vi "Q14070Z130主界面.vi"() -> ()   [LabVIEW 2013]
panel:
  out "操作步骤":bool[](array[boolean])
  out "实际涂脂":i32 format="%.0g"
  out "涂脂频率":dbl
  out "涂脂次数":i32
  out "气缸压装":dbl
  out "塞头辅具":dbl
  out "定位辅具":dbl
  out "压装辅具":dbl
  out "拧紧信号":dbl
  out "涂脂启动":dbl
  out "螺栓取料":dbl
  out "弹垫取料":dbl
  out "防尘罩O型圈":dbl
  out "胶塞取料":dbl
  out "J728程序选择":bool
  out "涂脂阀2":bool
  out "涂脂阀1":bool
  out "涂脂按钮2":bool
  out "涂脂按钮1":bool
  out "启动1按钮":bool
  out "启动2按钮":bool
  out "压缸下压时间":dbl
  out "扫描条码完成":bool
  out "扫描条码触发":bool
  out "开始时间":string
  in  "结束时间":string
  in  "返工次数":i32
  out "J706程序选择":bool
  out "J709程序选择":bool
  in  "产品ID":string
  out "员工ID":string
  out "员工姓名":string
  out "参数保存错误":errorcluster
  in  "报警清除":bool
  in  "参数加载":bool
  in  "型号选择":u32(ring) items=["J706", "J709", "J728", "J728A", "J728B", "J506X"]
  out "参数加载错误":errorcluster
  in  "停止":bool
  out "ADODB._Connection Out":refnum<k7>
  out "参数查询错误":errorcluster
  in  "联线按钮":bool
  out "通讯状态":bool
  in  "选项卡控件":enum32{"自动界面", "物料批次号输入", "参数查询"}(tab)
  out "涂脂报警工步号":u32 caption="工步号1"
  out "自动工步提示 3":string
  out "J728工布号提示":string
  in  "J728工步号提示":i32
  in  "产品ID字符位数":dbl
  in  "批次号工步号":u32=5 caption="工步号1"
  out "压装辅具在位":bool
  out "定位辅具在位":bool
  out "塞头辅具在位":bool
  out "记号笔在位":bool
  out "取压装辅具指示灯":bool
  out "取定位辅具指示灯":bool
  out "取塞头辅具指示灯":bool
  out "取记号笔指示灯":bool
  out "涂脂阀3":bool
  out "绿灯":bool
  out "黄灯":bool
  out "红灯":bool
  out "涂脂按钮3":bool
  in  "J709工步号提示":u32 caption="工步号1"
  out "自动工步提示 2":string
  out "自动工步号":u32 caption="工步号1"
  in  "报警工步号":u32 caption="工步号1"
  out "自动工步提示":string
  out "报警提示":string
  out "安全光幕":bool
  out "急停按钮":bool
  out "复位按钮":bool
  out "手动/自动":bool
  in  "压装气缸下降":bool
  in  "压装气缸上升":bool
  out "压装气缸上位检测":bool
  out "压装气缸下位检测":bool
  out "压装气缸下压阀":bool
  out "上序合格":bool
  out "上序完成":bool
  out "本序完成":bool
  out "本序合格":bool
  in  "装防尘罩循环启动":bool
  out "批次号提示":string
  in  "弹垫批次号位数":dbl
  in  "花键套批次号位数":dbl
  in  "胶塞批次号位数":dbl
  in  "螺栓批次号位数":dbl
  in  "防尘罩批次号位数":dbl
  out "弹垫批次号输入成功":bool
  out "花键套批次号输入成功":bool
  out "胶塞批次号输入成功":bool
  out "螺栓批次号输入成功":bool
  out "防尘罩批次号输入成功":bool
  in  "弹垫批次号":string
  in  "花键套批次号":string
  in  "胶塞批次号":string
  in  "螺栓批次号":string
  in  "防尘罩批次号":string
  in  "参数保存":bool
  in  "参数查询":bool
  in  "参数列表":string[][](table)
  # "装防尘罩"
  # "Copying (C) 2015 湖北唯思凌科装备制造有限公司 版权所有"
  # "输入成功"
  # "批次号位数"
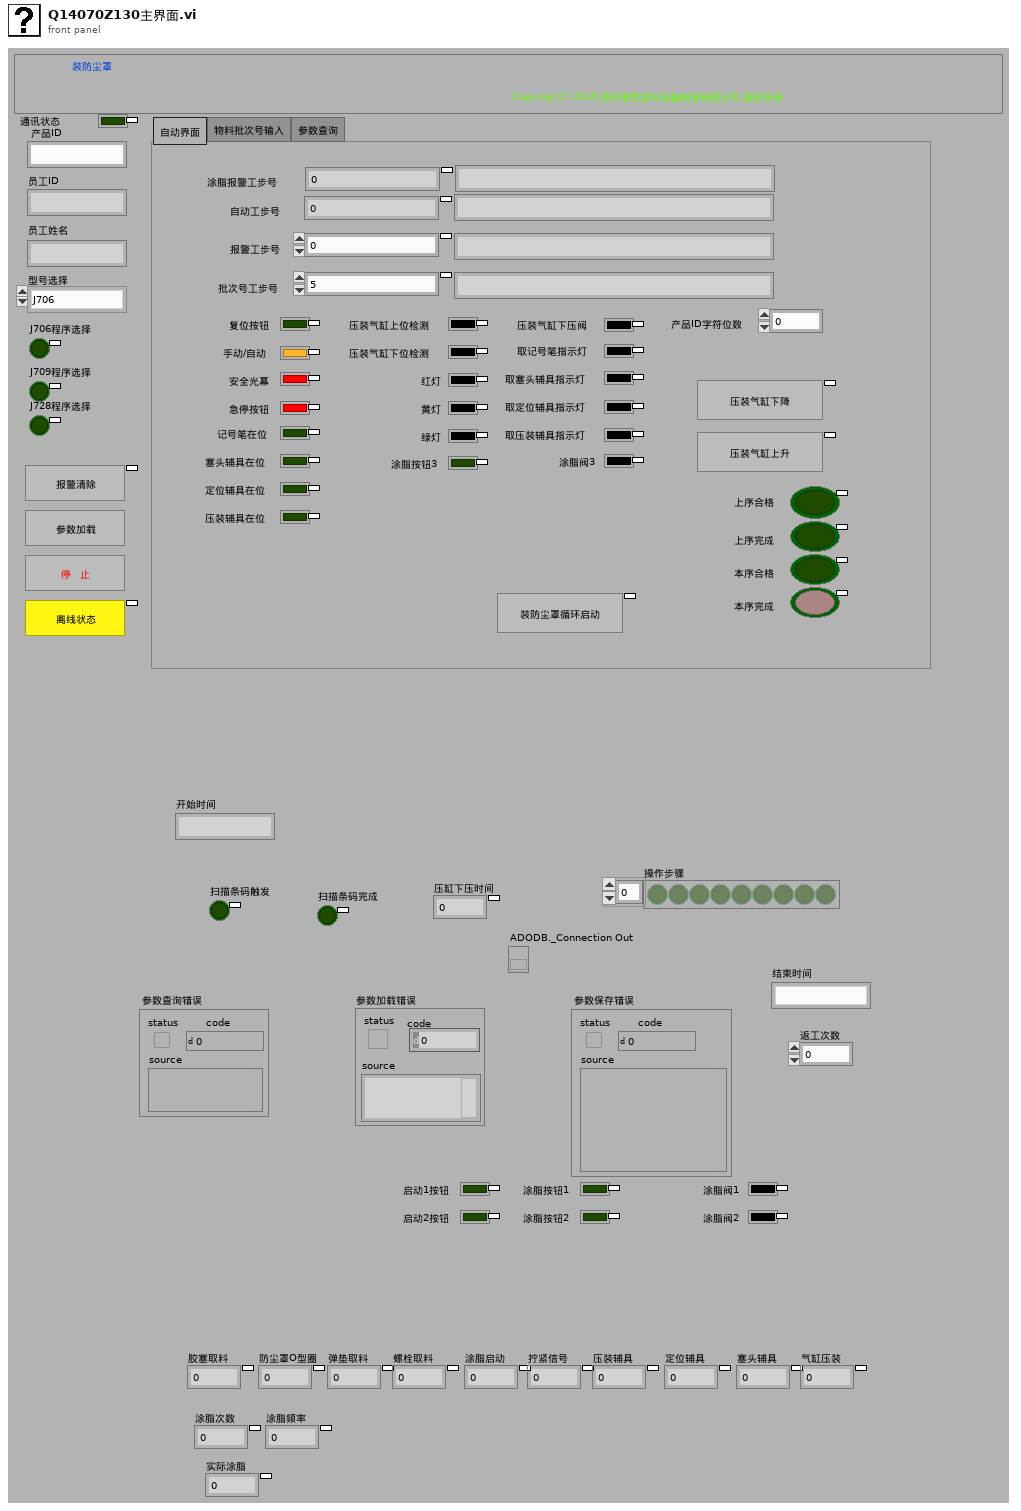
[diagram p1: front panel]
types:
  T1 = enum32{"invalid app kind", "Development System", "Run Time System", "Student Edition", "Embedded LabVIEW", "Evaluation", "Custom"}
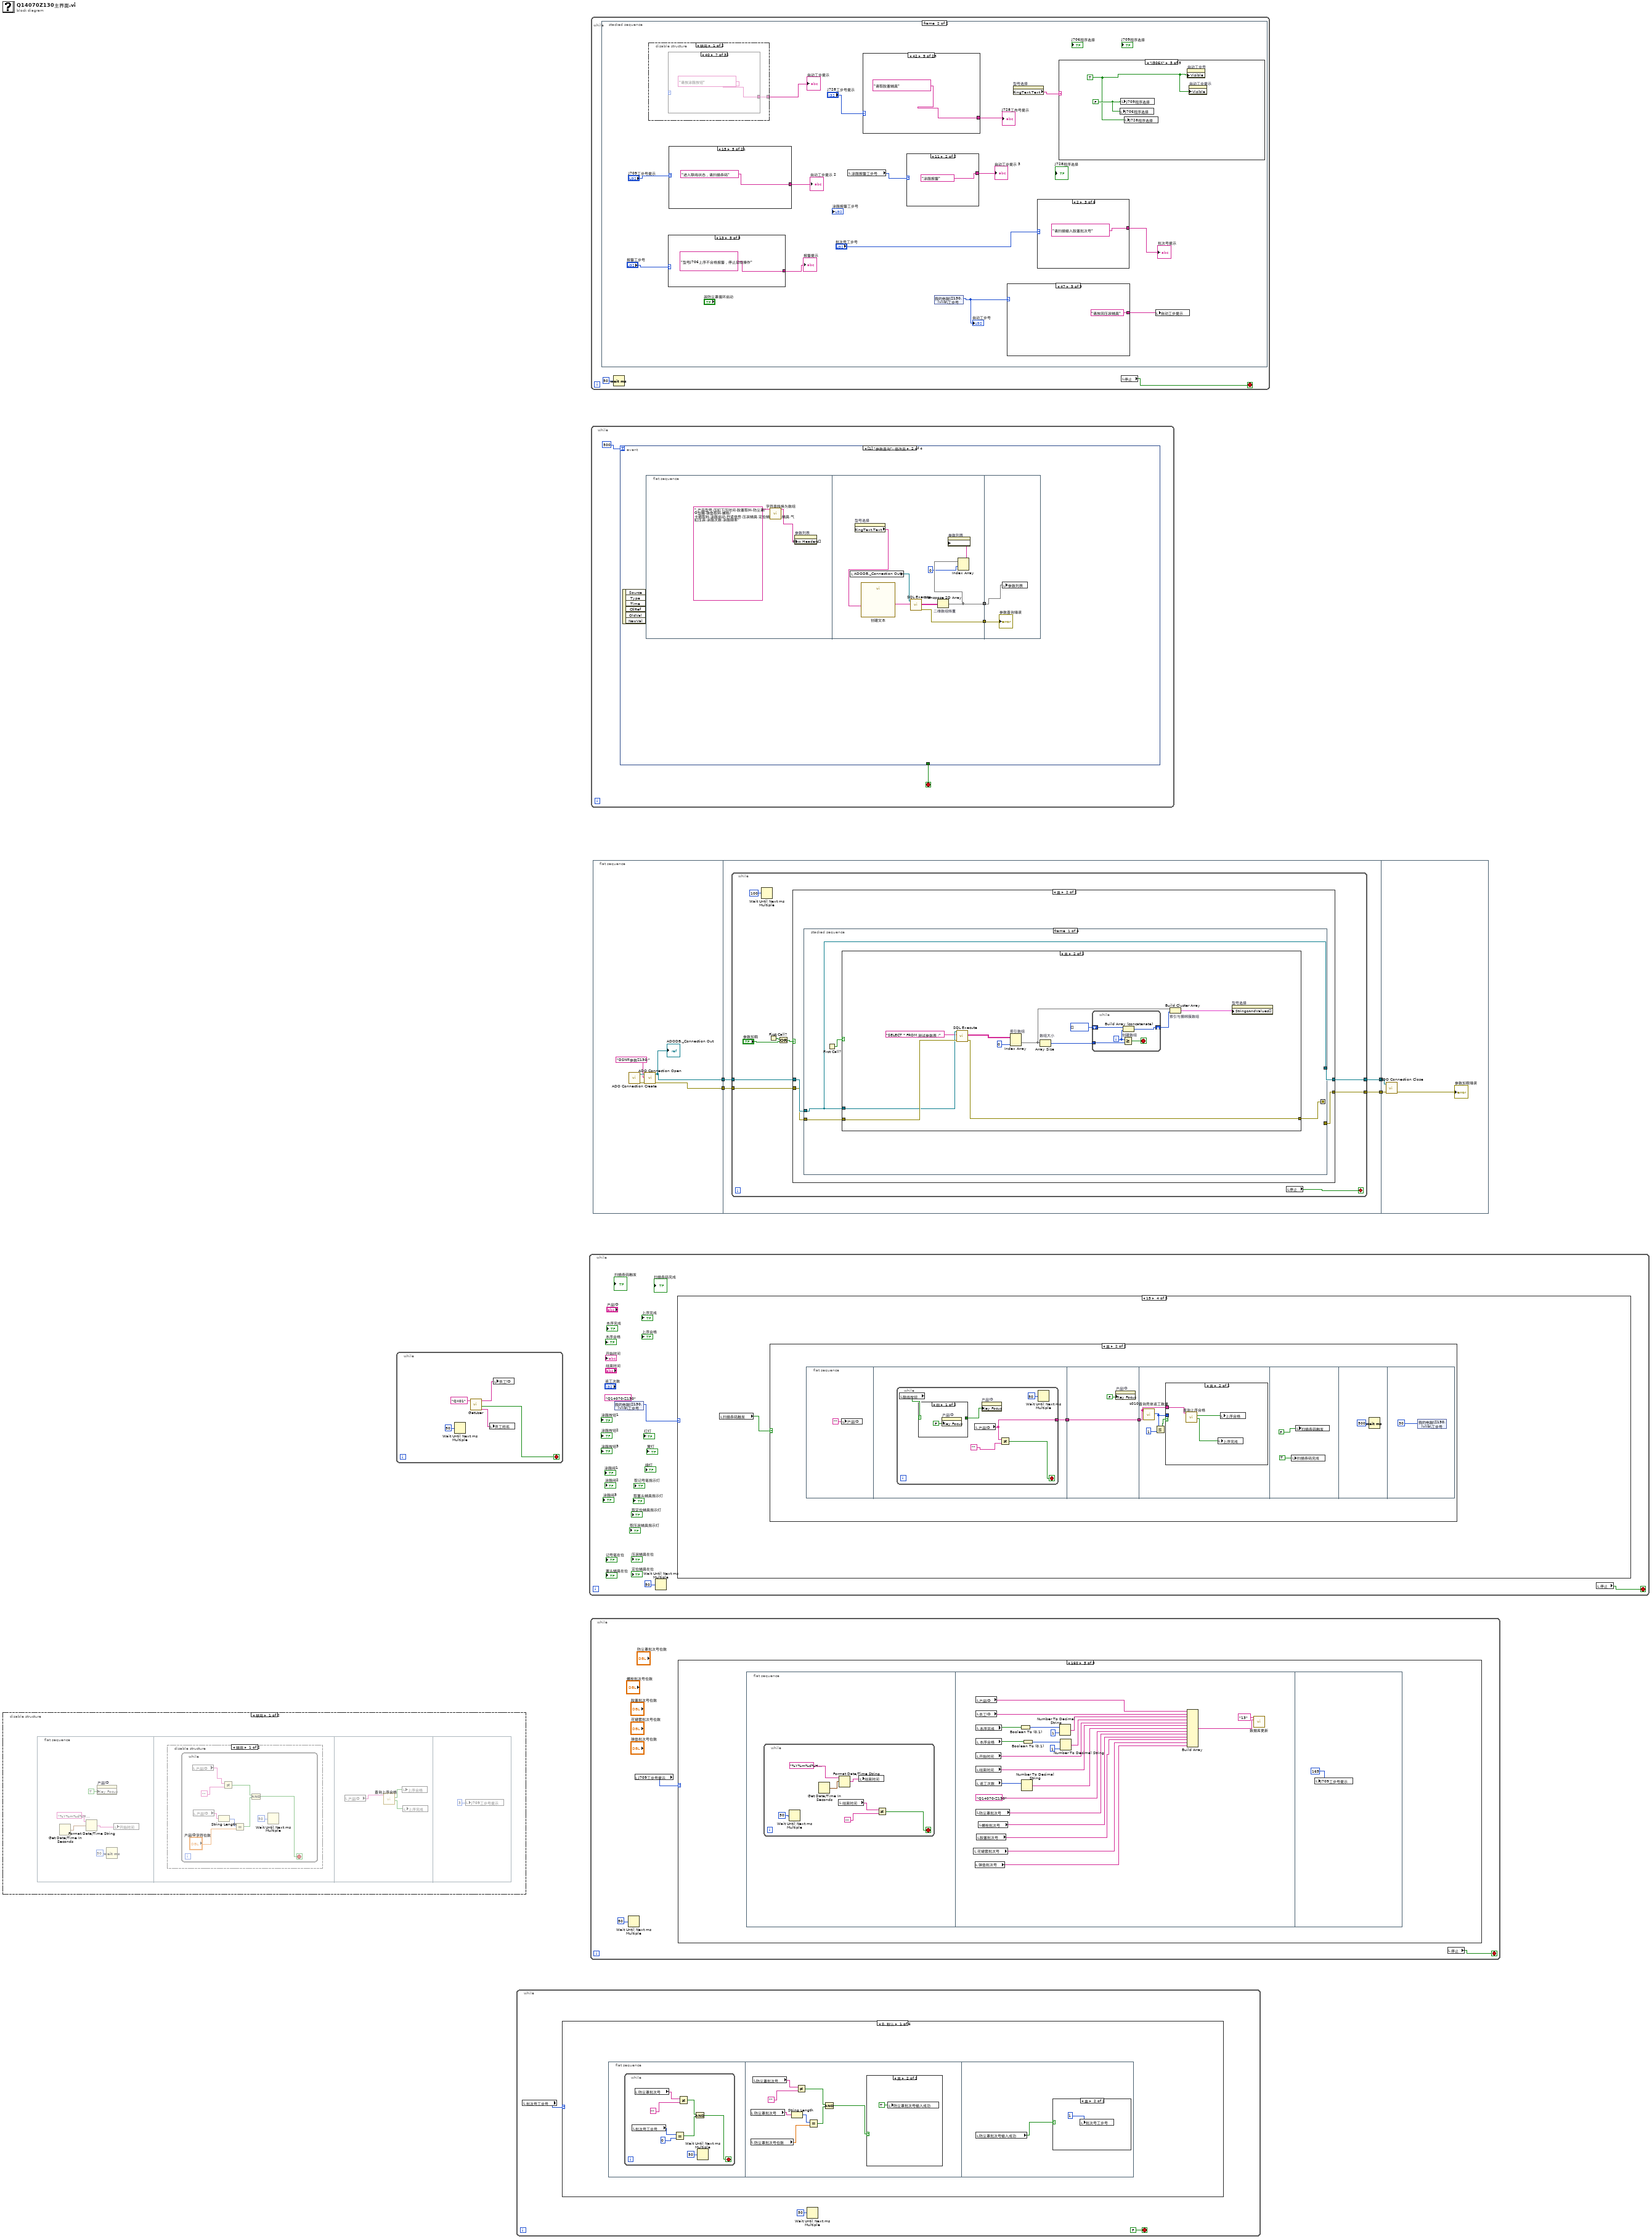
[diagram p0: block diagram]
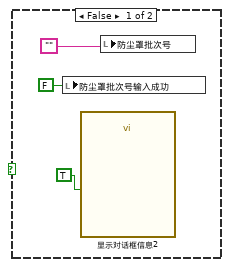
[diagram p4: hidden frame]
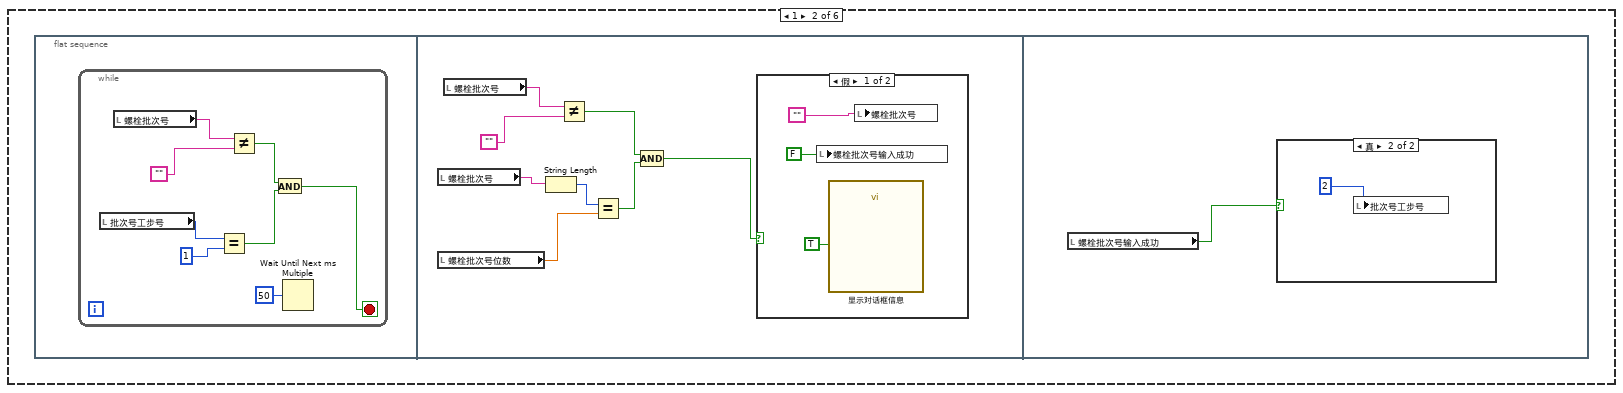
[diagram p6: hidden frame]
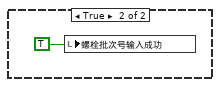
[diagram p7: hidden frame]
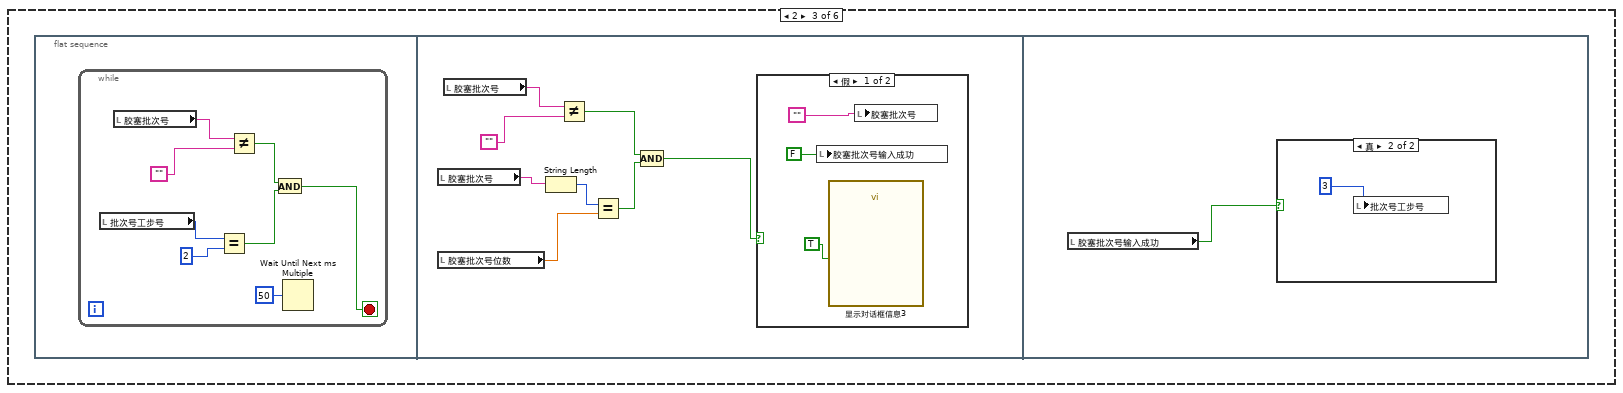
[diagram p9: hidden frame]
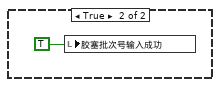
[diagram p10: hidden frame]
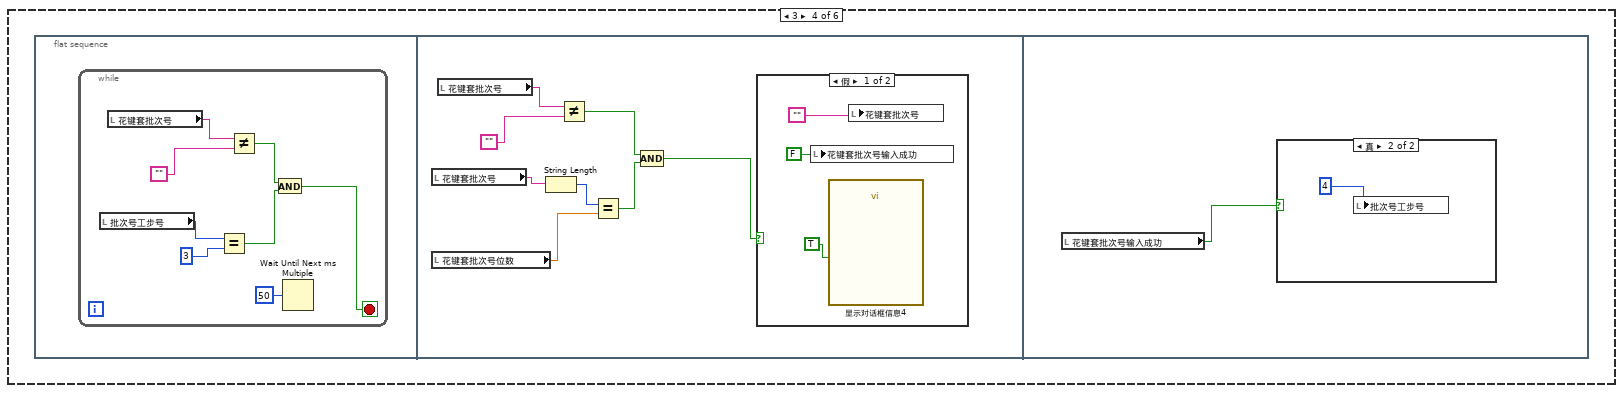
[diagram p12: hidden frame]
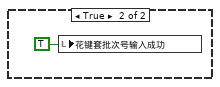
[diagram p13: hidden frame]
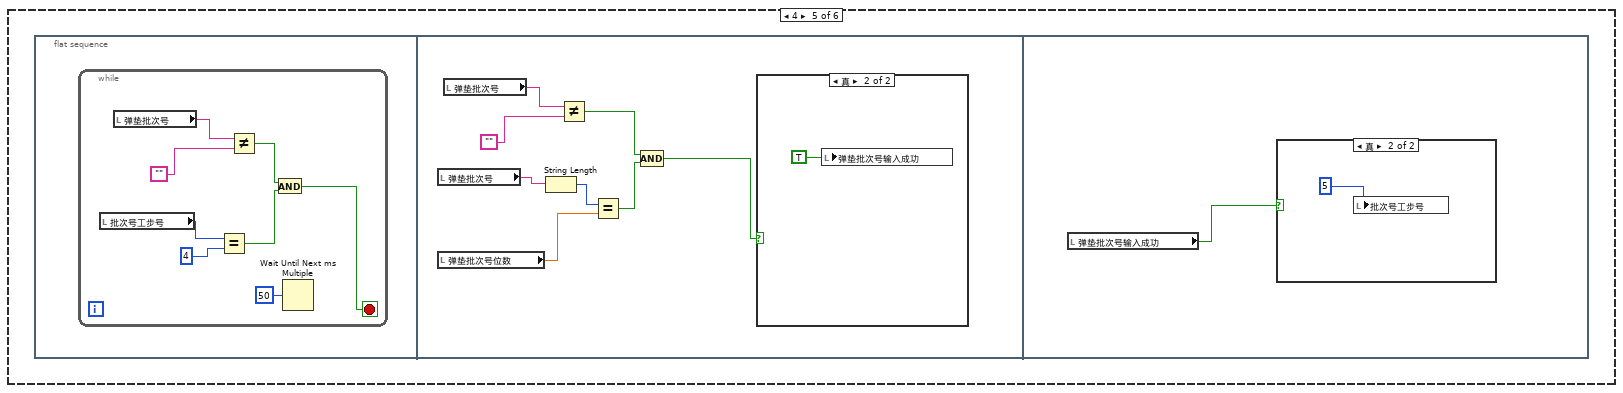
[diagram p15: hidden frame]
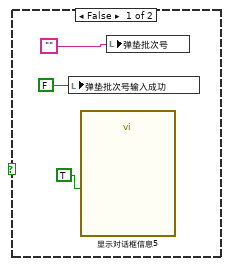
[diagram p16: hidden frame]
diagram:
  n1 = disable-structure shown="禁用" {
    frame Disabled {
      n2 = flat-sequence {
        frame #0 {
          n3 = Get Date/Time In Seconds() -> (seconds since 1Jan1904=w8:timestamp)
          n4 = Format Date/Time String(time format string (%c)="%Y%m%d%H%M" ("时间格式字符串(%c)"), seconds (now)=w8) -> (date/time string=w6:string)  [unwired: 1 in]
          n5 = property on="产品ID" class="Str"("Key Focus"=TRUE ("键选中")) -> ()  [unwired: 2 in, 2 out]
          n6 = Wait (ms)(milliseconds to wait=u32 50 ("等待时间（毫秒）")) -> ()  [unwired: 1 out]
          n7 = local write "开始时间"(w6) -> ()
        }
        frame #1 {
          n8 = disable-structure shown="禁用" {
            frame Disabled {
              n9 = while {
                stop <- w13 stop-if-true
                n10 = local read "产品ID"() -> (w10:string)
                n11 = local read "产品ID"() -> (w17:string)
                n12 = String Length(string=w17) -> (length=w16:i32)
                n13 = Not Equal?(x=w10, y="") -> (x != y?=w14:bool)
                n14 = Equal?(x=w16, y="产品ID字符位数") -> (x = y?=w15:bool)
                n15 = Compound Arithmetic op=AND(w14, w15) -> (w13:bool)
                n16 = Wait Until Next ms Multiple(millisecond multiple=u32 50 ("毫秒倍数")) -> ()  [unwired: 1 out]
              }
            }
            frame Enabled {
            }
          }
        }
        frame #2 {
          n17 = local read "产品ID"() -> (w21:string)
          n18 = call "查询上序合格.vi"("产品ID"=w21) -> ("本序已做"=w19:bool, "上序合格"=w20:bool)  [unwired: 8 in, 1 out]
          n19 = local write "上序合格"(w20) -> ()
          n20 = local write "上序完成"(w19) -> ()
        }
        frame #3 {
          n21 = local write "J709工步号提示"(u32 3 ("J709工步号提示")) -> ()
        }
      }
    }
    frame Enabled {
    }
  }
  n22 = while {
    stop <- w24 stop-if-true
    n23 = Wait Until Next ms Multiple(millisecond multiple=u32 50 ("毫秒倍数")) -> ()  [unwired: 1 out]
    n24 = call "GetUser.vi"("权限"="QX01") -> ("员工姓名"=w26:string, "权限"=w24:bool, "输入员工ID"=w25:string)  [unwired: 8 in]
    n25 = local write "员工姓名"(w26) -> ()
    n26 = local write "员工ID"(w25) -> ()
  }
  n27 = while {
    stop <- FALSE stop-if-true
    n28 = local read "批次号工步号"() -> (w30:u32)
    n29 = case shown="0, 默认" w30 {
      frame 0, Default {
        n30 = flat-sequence {
          frame #0 {
            n31 = while {
              stop <- w32 stop-if-true
              n32 = local read "批次号工步号"() -> (w36:u32)
              n33 = local read "防尘罩批次号"() -> (w38:string)
              n34 = Equal?(x=w36, y=u32 0) -> (x = y?=w33:bool)
              n35 = Not Equal?(x=w38, y="") -> (x != y?=w34:bool)
              n36 = And(x=w34, y=w33) -> (x .and. y?=w32:bool)
              n37 = Wait Until Next ms Multiple(millisecond multiple=u32 50 ("毫秒倍数")) -> ()  [unwired: 1 out]
            }
          }
          frame #1 {
            n38 = local read "防尘罩批次号"() -> (w46:string)
            n39 = local read "防尘罩批次号位数"() -> (w42:dbl)
            n40 = local read "防尘罩批次号"() -> (w44:string)
            n41 = String Length(string=w46) -> (length=w43:i32)
            n42 = Not Equal?(x=w44, y="") -> (x != y?=w41:bool)
            n43 = Equal?(x=w43, y=w42) -> (x = y?=w40:bool)
            n44 = Compound Arithmetic op=AND(w41, w40) -> (w39:bool)
            n45 = case shown="真" w39 {
              frame False {
                n46 = local write "防尘罩批次号输入成功"(FALSE ("防尘罩批次号输入成功")) -> ()
                n47 = call "显示对话框信息2"("Enable"=TRUE) -> ()  [unwired: 9 in, 2 out]
                n48 = local write "防尘罩批次号"("") -> ()
              }
              frame True {
                n49 = local write "防尘罩批次号输入成功"(TRUE ("防尘罩批次号输入成功")) -> ()
              }
            }
          }
          frame #2 {
            n50 = local read "防尘罩批次号输入成功"() -> (w51:bool)
            n51 = case shown="真" w51 {
              frame False {
              }
              frame True {
                n52 = local write "批次号工步号"(u32 1 ("报警工步号")) -> ()
              }
            }
          }
        }
      }
      frame 1 {
        n53 = flat-sequence {
          frame #0 {
            n54 = while {
              stop <- w54 stop-if-true
              n55 = local read "批次号工步号"() -> (w58:u32)
              n56 = local read "螺栓批次号"() -> (w60:string)
              n57 = Equal?(x=w58, y=u32 1) -> (x = y?=w55:bool)
              n58 = Not Equal?(x=w60, y="") -> (x != y?=w56:bool)
              n59 = And(x=w56, y=w55) -> (x .and. y?=w54:bool)
              n60 = Wait Until Next ms Multiple(millisecond multiple=u32 50 ("毫秒倍数")) -> ()  [unwired: 1 out]
            }
          }
          frame #1 {
            n61 = local read "螺栓批次号"() -> (w68:string)
            n62 = local read "螺栓批次号位数"() -> (w64:dbl)
            n63 = local read "螺栓批次号"() -> (w66:string)
            n64 = String Length(string=w68) -> (length=w65:i32)
            n65 = Not Equal?(x=w66, y="") -> (x != y?=w63:bool)
            n66 = Equal?(x=w65, y=w64) -> (x = y?=w62:bool)
            n67 = Compound Arithmetic op=AND(w63, w62) -> (w61:bool)
            n68 = case shown="假" w61 {
              frame False {
                n69 = local write "螺栓批次号输入成功"(FALSE ("防尘罩批次号输入成功")) -> ()
                n70 = call "显示对话框信息"("Enable"=TRUE) -> ()  [unwired: 9 in, 2 out]
                n71 = local write "螺栓批次号"("") -> ()
              }
              frame True {
                n72 = local write "螺栓批次号输入成功"(TRUE ("防尘罩批次号输入成功")) -> ()
              }
            }
          }
          frame #2 {
            n73 = local read "螺栓批次号输入成功"() -> (w73:bool)
            n74 = case shown="真" w73 {
              frame False {
              }
              frame True {
                n75 = local write "批次号工步号"(u32 2 ("报警工步号")) -> ()
              }
            }
          }
        }
      }
      frame 2 {
        n76 = flat-sequence {
          frame #0 {
            n77 = while {
              stop <- w76 stop-if-true
              n78 = local read "批次号工步号"() -> (w80:u32)
              n79 = local read "胶塞批次号"() -> (w82:string)
              n80 = Equal?(x=w80, y=u32 2) -> (x = y?=w77:bool)
              n81 = Not Equal?(x=w82, y="") -> (x != y?=w78:bool)
              n82 = And(x=w78, y=w77) -> (x .and. y?=w76:bool)
              n83 = Wait Until Next ms Multiple(millisecond multiple=u32 50 ("毫秒倍数")) -> ()  [unwired: 1 out]
            }
          }
          frame #1 {
            n84 = local read "胶塞批次号"() -> (w90:string)
            n85 = local read "胶塞批次号位数"() -> (w86:dbl)
            n86 = local read "胶塞批次号"() -> (w88:string)
            n87 = String Length(string=w90) -> (length=w87:i32)
            n88 = Not Equal?(x=w88, y="") -> (x != y?=w85:bool)
            n89 = Equal?(x=w87, y=w86) -> (x = y?=w84:bool)
            n90 = Compound Arithmetic op=AND(w85, w84) -> (w83:bool)
            n91 = case shown="假" w83 {
              frame False {
                n92 = local write "胶塞批次号输入成功"(FALSE ("防尘罩批次号输入成功")) -> ()
                n93 = call "显示对话框信息3"("Enable"=TRUE) -> ()  [unwired: 9 in, 2 out]
                n94 = local write "胶塞批次号"("") -> ()
              }
              frame True {
                n95 = local write "胶塞批次号输入成功"(TRUE ("防尘罩批次号输入成功")) -> ()
              }
            }
          }
          frame #2 {
            n96 = local read "胶塞批次号输入成功"() -> (w95:bool)
            n97 = case shown="真" w95 {
              frame False {
              }
              frame True {
                n98 = local write "批次号工步号"(u32 3 ("报警工步号")) -> ()
              }
            }
          }
        }
      }
      frame 3 {
        n99 = flat-sequence {
          frame #0 {
            n100 = while {
              stop <- w98 stop-if-true
              n101 = local read "批次号工步号"() -> (w102:u32)
              n102 = local read "花键套批次号"() -> (w104:string)
              n103 = Equal?(x=w102, y=u32 3) -> (x = y?=w99:bool)
              n104 = Not Equal?(x=w104, y="") -> (x != y?=w100:bool)
              n105 = And(x=w100, y=w99) -> (x .and. y?=w98:bool)
              n106 = Wait Until Next ms Multiple(millisecond multiple=u32 50 ("毫秒倍数")) -> ()  [unwired: 1 out]
            }
          }
          frame #1 {
            n107 = local read "花键套批次号"() -> (w112:string)
            n108 = local read "花键套批次号位数"() -> (w108:dbl)
            n109 = local read "花键套批次号"() -> (w110:string)
            n110 = String Length(string=w112) -> (length=w109:i32)
            n111 = Not Equal?(x=w110, y="") -> (x != y?=w107:bool)
            n112 = Equal?(x=w109, y=w108) -> (x = y?=w106:bool)
            n113 = Compound Arithmetic op=AND(w107, w106) -> (w105:bool)
            n114 = case shown="假" w105 {
              frame False {
                n115 = local write "花键套批次号输入成功"(FALSE ("防尘罩批次号输入成功")) -> ()
                n116 = call "显示对话框信息4"("Enable"=TRUE) -> ()  [unwired: 9 in, 2 out]
                n117 = local write "花键套批次号"("") -> ()
              }
              frame True {
                n118 = local write "花键套批次号输入成功"(TRUE ("防尘罩批次号输入成功")) -> ()
              }
            }
          }
          frame #2 {
            n119 = local read "花键套批次号输入成功"() -> (w117:bool)
            n120 = case shown="真" w117 {
              frame False {
              }
              frame True {
                n121 = local write "批次号工步号"(u32 4 ("报警工步号")) -> ()
              }
            }
          }
        }
      }
      frame 4 {
        n122 = flat-sequence {
          frame #0 {
            n123 = while {
              stop <- w120 stop-if-true
              n124 = local read "批次号工步号"() -> (w124:u32)
              n125 = local read "弹垫批次号"() -> (w126:string)
              n126 = Equal?(x=w124, y=u32 4) -> (x = y?=w121:bool)
              n127 = Not Equal?(x=w126, y="") -> (x != y?=w122:bool)
              n128 = And(x=w122, y=w121) -> (x .and. y?=w120:bool)
              n129 = Wait Until Next ms Multiple(millisecond multiple=u32 50 ("毫秒倍数")) -> ()  [unwired: 1 out]
            }
          }
          frame #1 {
            n130 = local read "弹垫批次号"() -> (w134:string)
            n131 = local read "弹垫批次号位数"() -> (w130:dbl)
            n132 = local read "弹垫批次号"() -> (w132:string)
            n133 = String Length(string=w134) -> (length=w131:i32)
            n134 = Not Equal?(x=w132, y="") -> (x != y?=w129:bool)
            n135 = Equal?(x=w131, y=w130) -> (x = y?=w128:bool)
            n136 = Compound Arithmetic op=AND(w129, w128) -> (w127:bool)
            n137 = case shown="真" w127 {
              frame False {
                n138 = local write "弹垫批次号输入成功"(FALSE ("防尘罩批次号输入成功")) -> ()
                n139 = call "显示对话框信息5"("Enable"=TRUE) -> ()  [unwired: 9 in, 2 out]
                n140 = local write "弹垫批次号"("") -> ()
              }
              frame True {
                n141 = local write "弹垫批次号输入成功"(TRUE ("防尘罩批次号输入成功")) -> ()
              }
            }
          }
          frame #2 {
            n142 = local read "弹垫批次号输入成功"() -> (w139:bool)
            n143 = case shown="真" w139 {
              frame False {
              }
              frame True {
                n144 = local write "批次号工步号"(u32 5 ("报警工步号")) -> ()
              }
            }
          }
        }
      }
      frame 5 {
      }
    }
    n145 = Wait Until Next ms Multiple(millisecond multiple=u32 50 ("毫秒倍数")) -> ()  [unwired: 1 out]
  }
  n146 = while {
    stop <- w142 stop-if-true
    (unwired) "Q14070-Z130"
    n147 = shared-variable "我的电脑\\Z130.lvlib\\工步号"() -> (w141:u16)  [unwired: 1 in, 1 out]
    n148 = Wait Until Next ms Multiple(millisecond multiple=u32 50 ("毫秒倍数")) -> ()  [unwired: 1 out]
    n149 = case shown="15" w141 {
      frame 0, Default {
      }
      frame 1 {
      }
      frame 5 {
        n150 = flat-sequence {
          frame #0 {
            n151 = while {
              stop <- w145 stop-if-true
              n152 = Get Date/Time In Seconds() -> (seconds since 1Jan1904=w149:timestamp)
              n153 = Wait (ms)(milliseconds to wait=u32 100 ("毫秒倍数")) -> ()  [unwired: 1 out]
              n154 = Format Date/Time String(time format string (%c)="%Y%m%d%H%M" ("时间格式字符串(%c)"), seconds (now)=w149) -> (date/time string=w148:string)  [unwired: 1 in]
              n155 = local read "开始时间"() -> (w147:string)
              n156 = local write "开始时间"(w148) -> ()
              n157 = Not Equal?(x=w147, y="") -> (x != y?=w145:bool)
            }
          }
          frame #1 {
            n158 = shared-variable "我的电脑\\Z130.lvlib\\工步号"(10 ("内球节工步号")) -> ()  [unwired: 1 in, 1 out]
          }
        }
      }
      frame 15 {
        n159 = local read "扫描条码触发"() -> (w152:bool)
        n160 = case shown="真" w152 {
          frame False {
          }
          frame True {
            n161 = flat-sequence {
              tunnel: [w156] -> w154
              tunnel: w154 -> [w165]
              tunnel: [w165] -> w153
              tunnel: w153 -> [w168]
              frame #0 {
                n162 = local write "产品ID"("" ("产品ID")) -> ()
              }
              frame #1 {
                n163 = while {
                  tunnel: [w159] -> w156
                  stop <- w160 stop-if-true
                  n164 = local read "联线按钮"() -> (w157:bool)
                  n165 = case shown="假" w157 {
                    tunnel: [_ TRUE ("键选中")] -> w158
                    frame False {
                      n166 = property on="产品ID" class="Str"("Key Focus"=FALSE ("键选中")) -> ()  [unwired: 2 in, 2 out]
                    }
                    frame True {
                    }
                  }
                  n167 = local read "产品ID"() -> (w159:string)
                  n168 = property on="产品ID" class="Str"("Key Focus"=w158) -> ()  [unwired: 2 in, 2 out]
                  n169 = Not Equal?(x=w159, y="") -> (x != y?=w160:bool)
                  n170 = Wait Until Next ms Multiple(millisecond multiple=u32 50 ("毫秒倍数")) -> ()  [unwired: 1 out]
                }
              }
              frame #2 {
                n171 = property on="产品ID" class="Str"("Key Focus"=FALSE ("键选中")) -> ()  [unwired: 2 in, 2 out]
              }
              frame #3 {
                n172 = call "z010查询壳体返工数量.vi"("转向器总成ID"=w168) -> ("Rows Fetched"=w167:i32)  [unwired: 8 in, 2 out]
                n173 = Less Or Equal?(x=w167, y=1) -> (x <= y?=w169:bool)
                n174 = case shown="真" w169 {
                  tunnel: w168 -> [w177 w180]
                  tunnel: w167 -> [w179 _]
                  frame False {
                    n175 = Subtract(x=w179, y=1) -> (x-y=w175:i32)
                    n176 = Number To Decimal String(number=w175) -> (decimal integer string=w174:string)  [unwired: 1 in]
                    n177 = Concatenate Strings(w177, "-" ("字符串"), w174) -> (w171:string)
                    n178 = call "查询上序合格.vi"("产品ID"=w171) -> ("本序已做"=w172:bool, "上序合格"=w173:bool)  [unwired: 8 in, 1 out]
                    n179 = local write "产品ID"(w171) -> ()
                    n180 = local write "上序完成"(w172) -> ()
                    n181 = local write "上序合格"(w173) -> ()
                  }
                  frame True {
                    n182 = call "查询上序合格.vi"("产品ID"=w180) -> ("本序已做"=w182:bool, "上序合格"=w181:bool)  [unwired: 8 in, 1 out]
                    n183 = local write "上序完成"(w182) -> ()
                    n184 = local write "上序合格"(w181) -> ()
                  }
                }
              }
              frame #4 {
                n185 = local write "扫描条码完成"(TRUE ("RFID读取完成-13")) -> ()
                n186 = local write "扫描条码触发"(FALSE ("RFID读取触发-13")) -> ()
              }
              frame #5 {
                n187 = Wait (ms)(milliseconds to wait=u32 500 ("等待时间（毫秒）")) -> ()  [unwired: 1 out]
              }
              frame #6 {
                n188 = shared-variable "我的电脑\\Z130.lvlib\\工步号"(30 ("内球节工步号")) -> ()  [unwired: 1 in, 1 out]
              }
            }
          }
        }
      }
      frame 140 {
        n189 = flat-sequence {
          frame #0 {
            n190 = while {
              stop <- w187 stop-if-true
              n191 = Wait Until Next ms Multiple(millisecond multiple=u32 50 ("毫秒倍数")) -> ()  [unwired: 1 out]
              n192 = Get Date/Time In Seconds() -> (seconds since 1Jan1904=w192:timestamp)
              n193 = local read "结束时间"() -> (w189:string)
              n194 = Format Date/Time String(time format string (%c)="%Y%m%d%H%M" ("时间格式字符串(%c)"), seconds (now)=w192) -> (date/time string=w193:string)  [unwired: 1 in]
              n195 = local write "结束时间"(w193) -> ()
              n196 = Not Equal?(x=w189, y="") -> (x != y?=w187:bool)
            }
          }
          frame #1 {
            n197 = local read "花键套批次号"() -> (w214:string)
            n198 = local read "弹垫批次号"() -> (w215:string)
            n199 = local read "产品ID"() -> (w202:string)
            n200 = local read "员工ID"() -> (w203:string)
            n201 = local read "开始时间"() -> (w206:string)
            n202 = local read "结束时间"() -> (w207:string)
            n203 = local read "防尘罩批次号"() -> (w211:string)
            n204 = local read "本序完成"() -> (w201:bool)
            n205 = local read "本序合格"() -> (w198:bool)
            n206 = local read "返工次数"() -> (w209:i32)
            n207 = local read "胶塞批次号"() -> (w213:string)
            n208 = local read "螺栓批次号"() -> (w212:string)
            n209 = Boolean To (0,1)(Boolean=w201) -> (0, 1=w199:i16)
            n210 = Number To Decimal String(number=w209) -> (decimal integer string=w210:string)  [unwired: 1 in]
            n211 = Boolean To (0,1)(Boolean=w198) -> (0, 1=w196:i16)
            n212 = Number To Decimal String(number=w199, width (-)=i16 1 ("宽度(-)")) -> (decimal integer string=w204:string)
            n213 = Number To Decimal String(number=w196, width (-)=i16 1 ("宽度(-)")) -> (decimal integer string=w205:string)
            n214 = Build Array(w202, w203, w204, w205, w206, w207, w210, "Q14070-Z130", w211, w212, w213, w214, w215) -> (w195:string[])
            n215 = call "数据库更新.vi"("设备号"="13", "数据"=w195) -> ()  [unwired: 13 in, 1 out]
          }
          frame #2 {
            n216 = Wait (ms)(milliseconds to wait=u32 2000 ("等待时间（毫秒）")) -> ()  [unwired: 1 out]
          }
          frame #3 {
            w217 = u16 145 ("工步号2")
            n217 = local write "J728工步号提示"(w217) -> ()
            n218 = local write "自动工步号"(w217) -> ()
          }
        }
      }
    }
    n219 = local read "停止"() -> (w142:bool)
  }
  n220 = while {
    stop <- w218 stop-if-true
    n221 = Wait Until Next ms Multiple(millisecond multiple=u32 50 ("毫秒倍数")) -> ()  [unwired: 1 out]
    n222 = local read "J709工步号提示"() -> (w220:u32)
    n223 = case shown="160" w220 {
      frame 0, Default {
      }
      frame 1 {
      }
      frame 5 {
        n224 = flat-sequence {
          frame #0 {
            n225 = while {
              stop <- w221 stop-if-true
              n226 = Wait Until Next ms Multiple(millisecond multiple=u32 50 ("毫秒倍数")) -> ()  [unwired: 1 out]
              n227 = Get Date/Time In Seconds() -> (seconds since 1Jan1904=w226:timestamp)
              n228 = Format Date/Time String(time format string (%c)="%Y%m%d%H%M" ("时间格式字符串(%c)"), seconds (now)=w226) -> (date/time string=w225:string)  [unwired: 1 in]
              n229 = local read "开始时间"() -> (w223:string)
              n230 = local write "开始时间"(w225) -> ()
              n231 = Not Equal?(x=w223, y="") -> (x != y?=w221:bool)
            }
          }
          frame #1 {
            n232 = local write "J709工步号提示"(10.0 ("内球节工步号")) -> ()
          }
        }
      }
      frame 15 {
        n233 = local read "扫描条码触发"() -> (w229:bool)
        n234 = case shown="真" w229 {
          frame False {
          }
          frame True {
            n235 = flat-sequence {
              tunnel: [w231] -> w230
              tunnel: w230 -> [w239]
              frame #0 {
                n236 = while {
                  tunnel: [w233] -> w231
                  stop <- w234 stop-if-true
                  n237 = local read "产品ID"() -> (w233:string)
                  n238 = property on="产品ID" class="Str"("Key Focus"=TRUE ("键选中")) -> ()  [unwired: 2 in, 2 out]
                  n239 = Not Equal?(x=w233, y="") -> (x != y?=w234:bool)
                  n240 = Wait Until Next ms Multiple(millisecond multiple=u32 50 ("毫秒倍数")) -> ()  [unwired: 1 out]
                }
              }
              frame #1 {
                n241 = call "查询上序合格.vi"("产品ID"=w239) -> ("本序已做"=w237:bool, "上序合格"=w238:bool)  [unwired: 8 in, 1 out]
                n242 = local write "上序完成"(w237) -> ()
                n243 = local write "上序合格"(w238) -> ()
              }
              frame #2 {
                n244 = local write "扫描条码完成"(TRUE ("RFID读取完成-13")) -> ()
                n245 = local write "扫描条码触发"(FALSE ("RFID读取触发-13")) -> ()
              }
              frame #3 {
                n246 = Wait (ms)(milliseconds to wait=u32 500 ("等待时间（毫秒）")) -> ()  [unwired: 1 out]
              }
              frame #4 {
                n247 = local write "J709工步号提示"(30.0 ("内球节工步号")) -> ()
              }
            }
          }
        }
      }
      frame 160 {
        n248 = flat-sequence {
          frame #0 {
            n249 = while {
              stop <- w244 stop-if-true
              n250 = Wait Until Next ms Multiple(millisecond multiple=u32 50 ("毫秒倍数")) -> ()  [unwired: 1 out]
              n251 = Get Date/Time In Seconds() -> (seconds since 1Jan1904=w249:timestamp)
              n252 = local read "结束时间"() -> (w246:string)
              n253 = Format Date/Time String(time format string (%c)="%Y%m%d%H%M" ("时间格式字符串(%c)"), seconds (now)=w249) -> (date/time string=w250:string)  [unwired: 1 in]
              n254 = local write "结束时间"(w250) -> ()
              n255 = Not Equal?(x=w246, y="") -> (x != y?=w244:bool)
            }
          }
          frame #1 {
            n256 = local read "花键套批次号"() -> (w254:string)
            n257 = local read "弹垫批次号"() -> (w253:string)
            n258 = local read "产品ID"() -> (w266:string)
            n259 = local read "员工ID"() -> (w265:string)
            n260 = local read "开始时间"() -> (w262:string)
            n261 = local read "结束时间"() -> (w261:string)
            n262 = local read "防尘罩批次号"() -> (w257:string)
            n263 = local read "本序完成"() -> (w267:bool)
            n264 = local read "本序合格"() -> (w270:bool)
            n265 = local read "返工次数"() -> (w259:i32)
            n266 = local read "胶塞批次号"() -> (w255:string)
            n267 = local read "螺栓批次号"() -> (w256:string)
            n268 = Boolean To (0,1)(Boolean=w267) -> (0, 1=w269:i16)
            n269 = Number To Decimal String(number=w259) -> (decimal integer string=w258:string)  [unwired: 1 in]
            n270 = Boolean To (0,1)(Boolean=w270) -> (0, 1=w272:i16)
            n271 = Number To Decimal String(number=w269, width (-)=i16 1 ("宽度(-)")) -> (decimal integer string=w264:string)
            n272 = Number To Decimal String(number=w272, width (-)=i16 1 ("宽度(-)")) -> (decimal integer string=w263:string)
            n273 = Build Array(w266, w265, w264, w263, w262, w261, w258, "Q14070-Z130", w257, w256, w255, w254, w253) -> (w252:string[])
            n274 = call "数据库更新.vi"("设备号"="13", "数据"=w252) -> ()  [unwired: 13 in, 1 out]
          }
          frame #2 {
            n275 = local write "J709工步号提示"(u16 165 ("工步号2")) -> ()
          }
        }
      }
    }
    n276 = local read "停止"() -> (w218:bool)
  }
  n277 = while {
    stop <- w274 stop-if-true
    n278 = event shown="[1] \"参数查询\": 值改变" {
      selector: _ -> [_ _ _ _]
      dyn-events: _ -> [_ _ _ _]
      timeout: 500 -> [_ _ _ _]
      tunnel: [_ _ _ w331] -> w274
      event Timeout {
        n279 = event-data() -> ()  [unwired: 1 in, 3 out]
      }
      event "参数查询": Value Change {
        n280 = event-data() -> ()  [unwired: 1 in, 6 out]
        n281 = flat-sequence {
          tunnel: [w285] -> w277
          tunnel: [w284] -> w276
          tunnel: w277 -> [w289]
          tunnel: w276 -> [w288]
          frame #0 {
            n282 = call "字符串转换为数组.vi"("查询内容"=",产品型号,压缸下压时间,胶塞取料,防尘罩/O型圈,弹垫取料,螺栓/卡箍取料,涂脂启动,拧紧信号,压装辅具,定位辅具,塞头辅具,气缸压装,涂脂次数,涂脂频率") -> ("列首"=w278:string[])  [unwired: 10 in]
            n283 = property on="参数列表" class="Tbl (严格)"("Row Headers[]"=w278) -> ()  [unwired: 2 in, 2 out]
          }
          frame #1 {
            n284 = local read "ADODB._Connection Out"() -> (w286:refnum<k7>)
            n285 = property on="型号选择" class="Ring (严格)"() -> ("RingText.Text"=w280:string)  [unwired: 2 in, 2 out]
            n286 = call "创建文本"("产品型号"=w280) -> ("Result"=w281:string)  [unwired: 13 in, 1 out]
            n287 = call "SQL Execute.vi"("Command Text"=w281, "ADODB._Connection In"=w286) -> ("error out"=w285:errorcluster, "Data"=w287:string[][])  [unwired: 6 in, 2 out]
            n288 = Transpose 2D Array "二维数组转置"(2D array=w287) -> (transposed array=w284:string[][])
            n289 = Index Array(array=w284, index (row)=0 ("禁用的索引 (列)")) -> (element=w283:string[])  [unwired: 1 in]
            n290 = property on="参数列表" class="Tbl (严格)"("Column Headers[]"=w283) -> ()  [unwired: 2 in, 2 out]
          }
          frame #2 {
            n291 = local write "参数列表"(w288) -> ()
            "参数查询错误" <- w289
          }
        }
      }
      event "参数保存": Value Change {
        n292 = event-data() -> ()  [unwired: 1 in, 6 out]
        n293 = while {
          i -> [w325]
          stop <- w327 stop-if-true
          n294 = local read "参数列表"() -> (w315:string[][])
          n295 = Greater Or Equal?(x=w325, y=2) -> (x >= y?=w327:bool)
          n296 = Index Array "索引数组"(array=w315, index (col)=w325) -> (element=w316:string[])  [unwired: 1 in]
          n297 = Index Array "索引数组"(array=w316, index=0 ("索引")) -> (element=w292:string)
          n298 = Wait Until Next ms Multiple(millisecond multiple=u32 100 ("毫秒倍数")) -> ()  [unwired: 1 out]
          n299 = Index Array(array=w316, index #1=1 ("索引"), index #2=2 ("索引"), index #3=3 ("索引"), index #4=4 ("索引"), index #5=5 ("索引"), index #6=6 ("索引"), index #7=7 ("索引"), index #8=8 ("索引"), index #9=9 ("索引"), index #10=10 ("索引"), index #11=11 ("索引")) -> (element #1=w303:string, element #2=w302:string, element #3=w301:string, element #4=w300:string, element #5=w299:string, element #6=w298:string, element #7=w297:string, element #8=w296:string, element #9=w295:string, element #10=w294:string, element #11=w293:string, element #12=w291:string, element #13=w290:string)  [unwired: 10 in, 8 out]
          n300 = call "创建文本3"("压缸下压时间"=w303, "胶塞取料"=w302, "防尘罩O型圈"=w301, "弹垫取料"=w300, "螺栓取料"=w299, "涂脂启动"=w298, "拧紧信号"=w297, "压装辅具"=w296, "定位辅具"=w295, "塞头辅具"=w294, "气缸压装"=w293, "涂脂次数"=w291, "涂脂频率"=w290, "产品型号"=w292) -> ("Result"=w304:string)  [unwired: 12 in, 1 out]
          n301 = call "ADO Connection Create.vi"() -> ("error out"=w321:errorcluster, "ADODB._Connection Out"=w322:refnum<k7>)  [unwired: 10 in]
          n302 = call "ADO Connection Open.vi"("error in (no error)"=w321, "ConnectionString"="DSN=参数Z130;", "ADODB._Connection In"=w322) -> ("error out"=w318:errorcluster, "ADODB._Connection Out"=w319:refnum<k7>)  [unwired: 7 in]
          n303 = call "SQL Execute.vi"("error in (no error)"=w318, "Command Text"=w304, "ADODB._Connection In"=w319) -> ("error out"=w328:errorcluster, "ADODB._Connection Out"=w329:refnum<k7>)  [unwired: 5 in, 2 out]
          n304 = call "ADO Connection Close.vi"("error in (no error)"=w328, "ADODB._Connection In"=w329) -> ("error out"=→"参数保存错误":errorcluster)  [unwired: 8 in, 1 out]
        }
      }
      event "停止": Value Change {
        n305 = event-data() -> ()  [unwired: 1 in, 6 out]
        n306 = property on="属性节点" class="App"() -> ("App.Kind"=w332:T1)  [unwired: 2 in, 2 out]
        n307 = case shown="\"Development System\"" w332 {
          tunnel: [_ w333 w334] -> w331
          frame "invalid app kind", Default {
          }
          frame "Development System" {
            w333 = TRUE ("停止？(T)")
            n308 = Stop(stop? (T)=w333) -> ()
          }
          frame "Run Time System" {
            w334 = TRUE ("退出？(T)")
            n309 = Quit LabVIEW(quit? (T)=w334) -> ()
          }
        }
      }
    }
  }
  n310 = while {
    stop <- w335 stop-if-true
    n311 = stacked-sequence {
      frame #0 {
      }
      frame #1 {
        n312 = disable-structure shown="禁用" {
          disable-tunnel: [w351 _] -> w343
          frame Disabled {
            n313 = case shown="40" {
              selector: _ -> [_ _ _ _ _ _ _ _ _ _ _ _ _ _ _ _ _ _ _ _ _ _ _ _ _ _ _ _ _ _ _ _]
              tunnel: ["工序开始,请扫描物料批次号" "工序开始,请点击装防尘罩循环启动" "工作开始，读取开始时间" "检查联线状态" "进入联线状态，请扫描条码" "扫描条码完成，根据上工序合格与否判断流程" "请按涂脂按钮" "请取胶塞" "请取胶塞" "请取胶塞辅具" "请取放回胶塞辅具" "请取定位辅具" "请放回定位辅具取压装辅具" "请双手启动" "气缸保压中" "请取防尘罩/O型圈" "请取螺栓/单耳无极卡箍" "请取弹垫" "请取扳手加力" "取料完成" "请放回压装辅具取密封垫" "胶塞安装完成后，请放回塞头辅具" "请取O型圈" "请取压装辅具" "请放回压装辅具" "双手启动" "保压中" "连线状态判断" "数据上传中" "数据上传完成，工位复位0" "型号J706上序不合格报警，停止后续操作" "数据上传"] -> w351
              frame 0, Default {
              }
              frame 1 {
              }
              frame 5 {
              }
              frame 10 {
              }
              frame 15 {
              }
              frame 30 {
              }
              frame 40 {
              }
              frame 41 {
              }
              frame 42 {
              }
              frame 43 {
              }
              frame 44 {
              }
              frame 45 {
              }
              frame 46 {
              }
              frame 50 {
              }
              frame 60 {
              }
              frame 70 {
              }
              frame 80 {
              }
              frame 90 {
              }
              frame 100 {
              }
              frame 120 {
              }
              frame 110 {
              }
              frame 130 {
              }
              frame 131 {
              }
              frame 132 {
              }
              frame 133 {
              }
              frame 136 {
              }
              frame 137 {
              }
              frame 138 {
              }
              frame 140 {
              }
              frame 145 {
              }
              frame 160 {
              }
              frame 165 {
              }
            }
          }
          frame Enabled {
          }
        }
        "自动工步提示" <- w343
        n314 = case shown="13" "报警工步号" {
          tunnel: ["工作正常" "急停被按下" "J709压装时压装时间过长 不回位" "型号J706上序不合格报警，停止后续操作" "型号J706上序不合格报警，停止后续操作"] -> w349
          frame 0, Default {
          }
          frame 10 {
          }
          frame 11 {
          }
          frame 12 {
          }
          frame 13 {
          }
        }
        "报警提示" <- w349
        n315 = case shown="15" "J709工步号提示" {
          tunnel: ["工序开始,请扫描物料批次号" "工序开始,请点击装防尘罩循环启动" "工作开始，读取开始时间" "检查联线状态 " "进入联线状态，请扫描条码" "扫描条码完成，根据上工序合格与否判断流程" "取防尘罩定位辅具" "防尘罩定位完毕后,双手启动进行压头压装" "压缸压装中，延迟2秒退回" "压缸回位后  取花键套 准备插入齿轮轴" "取螺栓" "取弹垫装到螺栓上，手工带扣" "用气缸定扭矩扳手 拧紧螺钉" "取记号笔做标记" "放回记号笔" "取胶塞" "取塞头辅具" "安装完成后，放回塞头辅具" "数据上传中" "数据上传完成，工位复位0" "型号J709上序不合格报警，停止后续操作"] -> w346
          frame 0, Default {
          }
          frame 1 {
          }
          frame 5 {
          }
          frame 10 {
          }
          frame 15 {
          }
          frame 30 {
          }
          frame 40 {
          }
          frame 50 {
          }
          frame 60 {
          }
          frame 70 {
          }
          frame 80 {
          }
          frame 90 {
          }
          frame 100 {
          }
          frame 110 {
          }
          frame 120 {
          }
          frame 130 {
          }
          frame 140 {
          }
          frame 150 {
          }
          frame 160 {
          }
          frame 165 {
          }
          frame 180 {
          }
        }
        "自动工步提示 2" <- w346
        n316 = local read "涂脂报警工步号"() -> (w340:u32)
        n317 = case shown="42" "J728工步号提示" {
          tunnel: ["工序开始,请扫描物料批次号" "工序开始,请点击装防尘罩循环启动" "工作开始，读取开始时间" "检查联线状态" "进入联线状态，请扫描条码" "扫描条码完成，根据上工序合格与否判断流程" "请按涂脂3按钮" "请取胶塞" "请取胶塞辅具" "请取防尘罩" "防尘罩置于涂脂辅具上后，启动涂脂3按钮" "请取胶塞 " "请取塞头辅具安装胶塞" "胶塞安装完成后，请放回塞头辅具" "请取O型圈" "请取压装辅具" "请放回压装辅具" "双手启动" "保压中" "连线状态判断" "数据上传中" "数据上传完成，工位复位0" "型号J706上序不合格报警，停止后续操作"] -> w341
          frame 0, Default {
          }
          frame 1 {
          }
          frame 5 {
          }
          frame 10 {
          }
          frame 15 {
          }
          frame 30 {
          }
          frame 40 {
          }
          frame 41 {
          }
          frame 42 {
          }
          frame 50 {
          }
          frame 60 {
          }
          frame 70 {
          }
          frame 120 {
          }
          frame 130 {
          }
          frame 131 {
          }
          frame 132 {
          }
          frame 133 {
          }
          frame 136 {
          }
          frame 137 {
          }
          frame 138 {
          }
          frame 140 {
          }
          frame 145 {
          }
          frame 160 {
          }
        }
        "J728工布号提示" <- w341
        n318 = case shown="11" w340 {
          tunnel: ["工作正常" "涂脂报警"] -> w339
          frame 0, Default {
          }
          frame 11 {
          }
        }
        "自动工步提示 3" <- w339
        n319 = shared-variable "我的电脑\\Z130.lvlib\\工步号"() -> (w337:u16)  [unwired: 1 in, 1 out]
        "自动工步号" <- w337
        n320 = case shown="47" w337 {
          tunnel: [_ "请按涂脂按钮3喷脂" "请取胶塞" "请取胶塞辅具" "请放回胶塞辅具" "请取压装辅具" "请双手启动，请勿触碰光幕" "压装保压中" "请放回压装辅具"] -> w338
          frame 0, Default {
          }
          frame 40 {
          }
          frame 41 {
          }
          frame 42 {
          }
          frame 43 {
          }
          frame 44 {
          }
          frame 45 {
          }
          frame 46 {
          }
          frame 47 {
          }
        }
        n321 = property on="型号选择" class="Ring (严格)"() -> ("RingText.Text"=w348:string)  [unwired: 2 in, 2 out]
        n322 = case shown="2" "批次号工步号" {
          tunnel: ["请扫描输入防尘罩批次号" "请扫描输入螺栓批次号" "请扫描输入胶塞批次号" "请扫描输入花键套批次号" "请扫描输入弹垫批次号" "批次号输入完毕，请开始工作"] -> w344
          frame 0, Default {
          }
          frame 1 {
          }
          frame 2 {
          }
          frame 3 {
          }
          frame 4 {
          }
          frame 5 {
          }
        }
        "批次号提示" <- w344
        n323 = case shown="\"J506X\"" w348 {
          frame "0", Default {
          }
          frame "J706" {
            w444 = FALSE ("程序选择-2")
            w445 = TRUE ("程序选择-1")
            n324 = local write "J728程序选择"(w444) -> ()
            n325 = local write "J706程序选择"(w445) -> ()
            n326 = local write "J709程序选择"(w444) -> ()
            n327 = property on="自动工步号" class="DigNum (严格)"("Visible"=w445) -> ()  [unwired: 2 in, 2 out]
            n328 = property on="自动工步提示" class="Str"("Visible"=w445) -> ()  [unwired: 2 in, 2 out]
          }
          frame "J709" {
            w446 = FALSE ("程序选择-2")
            w447 = TRUE ("程序选择-1")
            n329 = local write "J706程序选择"(w446) -> ()
            n330 = local write "J709程序选择"(w447) -> ()
            n331 = local write "J728程序选择"(w446) -> ()
            n332 = property on="自动工步号" class="DigNum (严格)"("Visible"=w447) -> ()  [unwired: 2 in, 2 out]
            n333 = property on="自动工步提示" class="Str"("Visible"=w447) -> ()  [unwired: 2 in, 2 out]
          }
          frame "J728" {
            w449 = FALSE ("程序选择-2")
            w448 = TRUE ("程序选择-1")
            n334 = local write "J706程序选择"(w449) -> ()
            n335 = local write "J709程序选择"(w449) -> ()
            n336 = local write "J728程序选择"(w448) -> ()
            n337 = property on="自动工步号" class="DigNum (严格)"("Visible"=w448) -> ()  [unwired: 2 in, 2 out]
            n338 = property on="自动工步提示" class="Str"("Visible"=w448) -> ()  [unwired: 2 in, 2 out]
          }
          frame "J506X" {
            w451 = FALSE ("程序选择-2")
            w450 = TRUE ("程序选择-1")
            n339 = local write "J706程序选择"(w451) -> ()
            n340 = local write "J709程序选择"(w451) -> ()
            n341 = local write "J728程序选择"(w450) -> ()
            n342 = property on="自动工步号" class="DigNum (严格)"("Visible"=w450) -> ()  [unwired: 2 in, 2 out]
            n343 = property on="自动工步提示" class="Str"("Visible"=w450) -> ()  [unwired: 2 in, 2 out]
          }
        }
        n344 = local write "自动工步提示"(w338) -> ()
      }
    }
    n345 = Wait (ms)(milliseconds to wait=u32 50 ("毫秒倍数")) -> ()  [unwired: 1 out]
    n346 = local read "停止"() -> (w335:bool)
  }
  n347 = flat-sequence {
    tunnel: [w457] -> w4
    tunnel: [w458] -> w3
    tunnel: w4 -> [w465]
    tunnel: w3 -> [w464]
    tunnel: [w463] -> w2
    tunnel: [w462] -> w1
    tunnel: w2 -> [w593]
    tunnel: w1 -> [w592]
    frame #0 {
      n348 = call "ADO Connection Create.vi"() -> ("error out"=w460:errorcluster, "ADODB._Connection Out"=w461:refnum<k7>)  [unwired: 10 in]
      n349 = call "ADO Connection Open.vi"("error in (no error)"=w460, "ConnectionString"="DSN=参数Z130;", "ADODB._Connection In"=w461) -> ("error out"=w458:errorcluster, "ADODB._Connection Out"=w457:refnum<k7>)  [unwired: 7 in]
      "ADODB._Connection Out" <- w457
    }
    frame #1 {
      n350 = while {
        tunnel: w465 -> [w474]
        tunnel: w464 -> [w473]
        tunnel: [w472] -> w463
        tunnel: [w471] -> w462
        stop <- w467 stop-if-true
        n351 = Wait Until Next ms Multiple(millisecond multiple=u32 100 ("毫秒倍数")) -> ()  [unwired: 1 out]
        n352 = First Call?() -> (First Call?: T/F=w470:bool)
        n353 = Or(x=w470, y="参数加载") -> (x .or. y?=w469:bool)
        n354 = case shown="真" w469 {
          tunnel: w474 -> [w476 w480]
          tunnel: w473 -> [w475 w479]
          tunnel: [w476 w478] -> w472
          tunnel: [w475 w477] -> w471
          frame False {
          }
          frame True {
            n355 = stacked-sequence {
              seq-local: [w482 _ _ _] -> [_ w533 _ _]
              tunnel: w480 -> [w483 w530 _ _]
              tunnel: w479 -> [w484 _ _ _]
              tunnel: [w483 _ _ _] -> w478
              tunnel: [_ w532 _ _] -> w477
              frame #0 {
                n356 = First Call?() -> (First Call?: T/F=w481:bool)
                n357 = case shown="真" w481 {
                  tunnel: w484 -> [w485 w496]
                  tunnel: w483 -> [_ w495]
                  tunnel: [w485 w494] -> w482
                  frame False {
                  }
                  frame True {
                    n358 = call "SQL Execute.vi"("error in (no error)"=w496, "Command Text"="SELECT * FROM 测试参数表 ;", "ADODB._Connection In"=w495) -> ("error out"=w494:errorcluster, "Data"=w488:string[][])  [unwired: 5 in, 2 out]
                    n359 = Index Array "索引数组"(array=w488, index (col)=0 ("禁用的索引 (列)")) -> (element=w491:string[])  [unwired: 1 in]
                    n360 = Array Size "数组大小"(array=w491) -> (size(s)=w490:i32)
                    n361 = while {
                      shift-right: [w499] -> w489
                      shift-left: i32[] [] -> [w500]
                      tunnel: w490 -> [w497]
                      i -> [w498]
                      stop <- w501 stop-if-true
                      n362 = Greater Or Equal?(x=w498, y=w497) -> (x >= y?=w501:bool)
                      n363 = Build Array (concatenate) "创建数组"(w500, w498) -> (w499:i32[])
                    }
                    n364 = Build Cluster Array "索引与捆绑簇数组"(w491, w489) -> (w486:cluster{"String":string, i32}[])
                    n365 = property on="型号选择" class="Ring (严格)"("StringsAndValues[]"=w486) -> ()  [unwired: 2 in, 2 out]
                  }
                }
              }
              frame #1 {
                n366 = property on="型号选择" class="Ring (严格)"() -> ("RingText.Text"=w528:string)  [unwired: 2 in, 2 out]
                n367 = call "创建文本4"("产品型号"=w528) -> ("Result"=w531:string)  [unwired: 13 in, 1 out]
                n368 = call "SQL Execute.vi"("error in (no error)"=w533, "Command Text"=w531, "ADODB._Connection In"=w530) -> ("error out"=w532:errorcluster, "Data"=w535:string[][])  [unwired: 5 in, 2 out]
                n369 = Index Array "索引数组"(array=w535, index (row)=0 ("索引 (行)")) -> (element=w529:string[])  [unwired: 1 in]
                n370 = Fract/Exp String To Number "分数/指数字符串至数值转换"(string=w529) -> (number=w527:dbl[])  [unwired: 3 in, 1 out]
                n371 = Index Array(array=w527, index #1=1 ("索引"), index #2=2 ("索引"), index #3=3 ("索引"), index #4=4 ("索引"), index #5=5 ("索引"), index #6=6 ("索引"), index #7=7 ("索引"), index #8=8 ("索引"), index #9=9 ("索引"), index #10=10 ("索引"), index #11=11 ("索引")) -> (element #1=→"压缸下压时间":dbl, element #2=→"胶塞取料":dbl, element #3=→"防尘罩O型圈":dbl, element #4=→"弹垫取料":dbl, element #5=→"螺栓取料":dbl, element #6=→"涂脂启动":dbl, element #7=→"拧紧信号":dbl, element #8=→"压装辅具":dbl, element #9=→"定位辅具":dbl, element #10=→"塞头辅具":dbl, element #11=→"气缸压装":dbl, element #12=→"涂脂次数":dbl, element #13=→"涂脂频率":dbl)  [unwired: 4 in, 2 out]
                "实际涂脂" <- 0 ("实际涂脂")
              }
              frame #2 {
                n372 = local read "ADODB._Connection Out"() -> (w540:refnum<k7>)
                n373 = call "SQL Execute.vi"("Command Text"="SELECT * FROM 传感器校验表 where ID='2'", "ADODB._Connection In"=w540) -> ("Data"=w541:string[][])  [unwired: 6 in, 3 out]
                n374 = Index Array "索引数组"(array=w541) -> (element=w542:string[])  [unwired: 2 in]
                n375 = Fract/Exp String To Number "分数/指数字符串至数值转换"(string=w542) -> (number=w543:dbl[])  [unwired: 3 in, 1 out]
                n376 = Index Array "索引数组"(array=w543, index #1=1 ("索引"), index #2=2 ("索引"), index #3=3 ("索引"), index #4=4 ("索引"), index #5=5 ("索引"), index #6=6 ("索引"), index #7=7 ("索引"), index #8=8 ("索引")) -> ()  [unwired: 8 out]
              }
              frame #3 {
                n377 = local read "胶塞取料"() -> (w571:dbl)
                n378 = local read "拧紧信号"() -> (w550:dbl)
                n379 = local read "防尘罩O型圈"() -> (w570:dbl)
                n380 = local read "螺栓取料"() -> (w569:dbl)
                n381 = local read "涂脂启动"() -> (w568:dbl)
                n382 = local read "弹垫取料"() -> (w551:dbl)
                n383 = local read "气缸压装"() -> (w564:dbl)
                n384 = local read "定位辅具"() -> (w566:dbl)
                n385 = local read "压装辅具"() -> (w567:dbl)
                n386 = local read "塞头辅具"() -> (w565:dbl)
                n387 = case shown="0, 默认" w568 {
                  tunnel: [FALSE TRUE] -> w559
                  frame 0, Default {
                  }
                  frame 1 {
                  }
                }
                n388 = case shown="0, 默认" w551 {
                  tunnel: [FALSE TRUE] -> w561
                  frame 0, Default {
                  }
                  frame 1 {
                  }
                }
                n389 = case shown="0, 默认" w569 {
                  tunnel: [FALSE TRUE] -> w560
                  frame 0, Default {
                  }
                  frame 1 {
                  }
                }
                n390 = case shown="0, 默认" w571 {
                  tunnel: [FALSE TRUE] -> w563
                  frame 0, Default {
                  }
                  frame 1 {
                  }
                }
                n391 = case shown="0, 默认" w564 {
                  tunnel: [FALSE TRUE] -> w554
                  frame 0, Default {
                  }
                  frame 1 {
                  }
                }
                n392 = case shown="0, 默认" w570 {
                  tunnel: [FALSE TRUE] -> w562
                  frame 0, Default {
                  }
                  frame 1 {
                  }
                }
                n393 = case shown="0, 默认" w550 {
                  tunnel: [FALSE TRUE] -> w558
                  frame 0, Default {
                  }
                  frame 1 {
                  }
                }
                n394 = case shown="0, 默认" w567 {
                  tunnel: [FALSE TRUE] -> w557
                  frame 0, Default {
                  }
                  frame 1 {
                  }
                }
                n395 = case shown="0, 默认" w565 {
                  tunnel: [FALSE TRUE] -> w555
                  frame 0, Default {
                  }
                  frame 1 {
                  }
                }
                n396 = case shown="0, 默认" w566 {
                  tunnel: [FALSE TRUE] -> w556
                  frame 0, Default {
                  }
                  frame 1 {
                  }
                }
                n397 = Build Array(w563, w562, w561, w560, w559, w558, w557, w556, w555, w554) -> (w553:bool[])
                n398 = Build Array (concatenate)(w553, bool[] [FALSE, FALSE, FALSE, FALSE, FALSE, FALSE]) -> (w549:bool[])
                "操作步骤" <- w549
                n399 = shared-variable "我的电脑\\Z130.lvlib\\QW3"(w549) -> ()  [unwired: 1 in, 1 out]
              }
            }
          }
        }
        n400 = local read "停止"() -> (w467:bool)
      }
    }
    frame #2 {
      n401 = call "ADO Connection Close.vi"("error in (no error)"=w592, "ADODB._Connection In"=w593) -> ("error out"=→"参数加载错误":errorcluster)  [unwired: 8 in, 1 out]
    }
  }
